vi "GetACK-NAK.vi"(0 "error in":errorcluster, 1 "Delay Time (s)":dbl) -> (2 "error out":errorcluster, 3 "Receive_buffer":u8[](array[numeric]), 4 "Status":bool)   [LabVIEW 2014]
panel:
  out "Read Time":u32
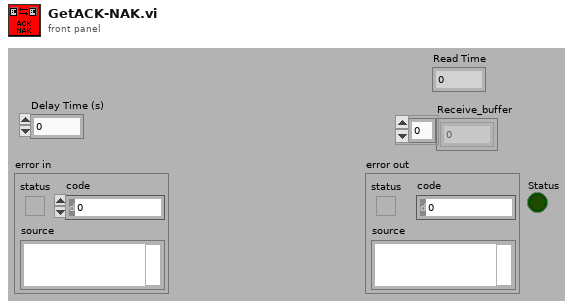
[diagram p1: front panel]
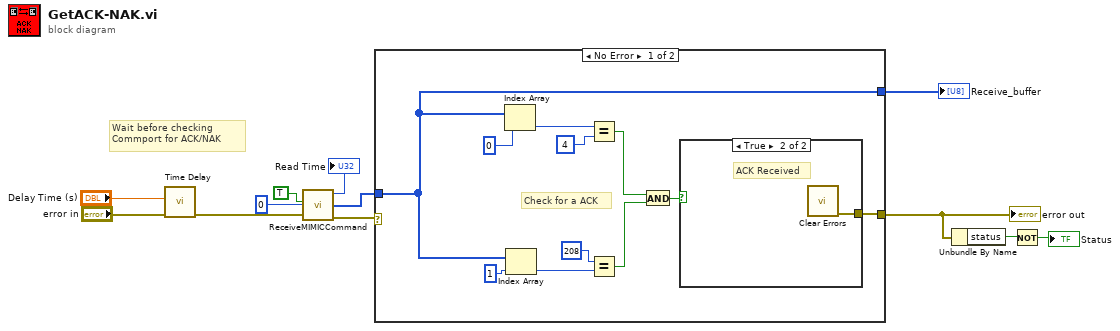
[diagram p0: block diagram]
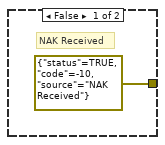
[diagram p2: hidden frame]
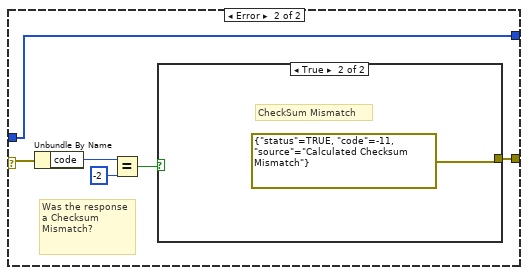
[diagram p3: hidden frame]
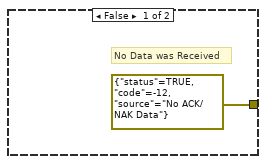
[diagram p4: hidden frame]
diagram:
  # "Wait before checking\nCommport for ACK/NAK"
  n1 = call "Time Delay"("error in (no error)"="error in", "Delay Time (s)"="Delay Time (s)") -> ("error out"=w4:errorcluster)  [unwired: 9 in]
  n2 = call "ReceiveMIMICCommand.vi"("error in"=w4, "Desired_Length"=u32 0, "CheckSum?"=TRUE) -> ("Receive_buffer"=w7:u8[], "error out"=w6:errorcluster, "Read Time"=→"Read Time":u32)  [unwired: 1 in, 2 out]
  n3 = case shown="No Error" w6 {
    selector: w6 -> [_ w30]
    tunnel: w7 -> [w13 w26]
    tunnel: [w14 w31] -> w12
    tunnel: [w13 w26] -> w9
    frame No Error {
      # "Check for a ACK"
      n4 = Index Array(array=w13, index=0) -> (element=w18:u8)
      n5 = Index Array(array=w13, index=1) -> (element=w17:u8)
      n6 = Equal?(x=w18, y=u8 4) -> (x = y?=w21:bool)
      n7 = Equal?(x=u8 208 ("y"), y=w17) -> (x = y?=w20:bool)
      n8 = And(x=w21, y=w20) -> (x .and. y?=w15:bool)
      n9 = case shown="True" w15 {
        tunnel: [errorcluster {"status"=TRUE, "code"=-10, "source"="NAK Received"} ("error out") w25] -> w14
        frame False {
          # "NAK Received"
        }
        frame True {
          # "ACK Received"
          n10 = call <vilib>:"Clear Errors.vi"() -> ("error out"=w25:errorcluster)  [unwired: 6 in, 1 out]
        }
      }
    }
    frame Error {
      # "Was the response a Checksum\nMismatch?"
      n11 = Unbundle By Name(w30) -> ("code"=w29:i32)
      n12 = Equal?(x=w29, y=-2) -> (x = y?=w27:bool)
      n13 = case shown="True" w27 {
        tunnel: [errorcluster {"status"=TRUE, "code"=-12, "source"="No ACK/NAK Data"} ("error out") errorcluster {"status"=TRUE, "code"=-11, "source"="Calculated Checksum Mismatch"} ("error out")] -> w31
        frame False {
          # "No Data was Received"
        }
        frame True {
          # "CheckSum Mismatch"
        }
      }
    }
  }
  "error out" <- w12
  "Receive_buffer" <- w9
  n14 = Unbundle By Name(w12) -> ("status"=w11:bool)
  n15 = Not(x=w11) -> (.not. x?=→"Status":bool)
